vi "Image_Standardize_Per_Channel(by_DS_Stats).vi"(7 "Dataset_Stats":T1={"means"={"R"=0.5385, "G"=0.5348, "B"=0.551}, "vars"={"R"=0.3673, "G"=0.3673, "B"=0.3505}, "DS_Size"=0} {"vars"."R" format="%#_3g"; "vars"."G" format="%#_3g"; "vars"."B" format="%#_3g"; "means"."R" format="%#_3g"; "means"."G" format="%#_3g"; "means"."B" format="%#_3g"}, 11 "In":sgl[][][](array[numeric])) -> (3 "Out":sgl[][][](array[numeric]))   [LabVIEW 2020]
uses:
  PatchCore_AddOn/API/Controls/NNPC_DS_Stats.ctl
  PatchCore_AddOn/API/Controls/Image_Stats_RGB.ctl
  PatchCore_AddOn/PatchCore_AddOn.lvlib
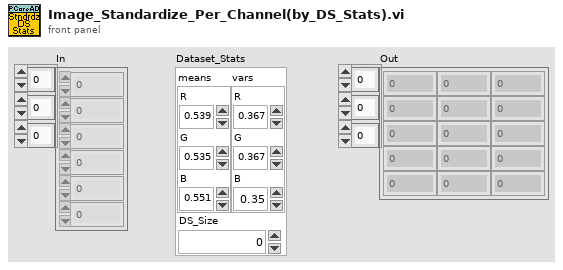
[diagram p1: front panel]
types:
  T1 = typedef "PatchCore_AddOn.lvlib/NNPC_DS_Stats.ctl" = cluster{"means":T2, "vars":T2, "DS_Size":i32}
  T2 = typedef "PatchCore_AddOn.lvlib/Image_Stats_RGB.ctl" = cluster{"R":sgl, "G":sgl, "B":sgl}
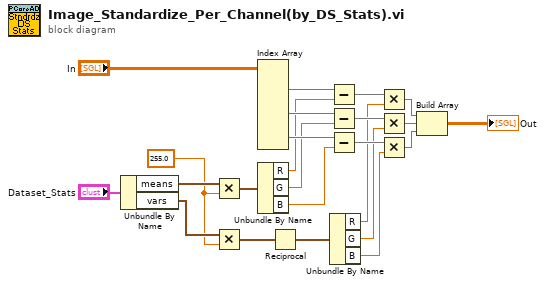
[diagram p0: block diagram]
diagram:
  w2 = sgl 255.0 ("R")
  n1 = Unbundle By Name("Dataset_Stats") -> ("means"=w7:T2, "vars"=w6:T2)
  n2 = Multiply(x=w7, y=w2) -> (x*y=w4:T2)
  n3 = Multiply(x=w6, y=w2) -> (x*y=w5:T2)
  n4 = Index Array(array="In") -> (element #1=w20:sgl[][], element #2=w19:sgl[][], element #3=w18:sgl[][])  [unwired: 9 in]
  n5 = Unbundle By Name(w4) -> ("R"=w13:sgl, "G"=w12:sgl, "B"=w11:sgl)
  n6 = Reciprocal(x=w5) -> (1/x=w1:T2)
  n7 = Subtract(x=w20, y=w13) -> (x-y=w24:sgl[][])
  n8 = Subtract(x=w19, y=w12) -> (x-y=w23:sgl[][])
  n9 = Subtract(x=w18, y=w11) -> (x-y=w22:sgl[][])
  n10 = Unbundle By Name(w1) -> ("R"=w10:sgl, "G"=w9:sgl, "B"=w8:sgl)
  n11 = Multiply(x=w24, y=w10) -> (x*y=w17:sgl[][])
  n12 = Multiply(x=w23, y=w9) -> (x*y=w16:sgl[][])
  n13 = Multiply(x=w22, y=w8) -> (x*y=w15:sgl[][])
  n14 = Build Array(w17, w16, w15) -> (→"Out":sgl[][][])
